vi "DOE Kitchen Data.vi"(6 "Data Logger Type":T1=enum."Agilent", 8 "Error In":errorcluster, 10 "Extra Data":dbl[](array[numeric]), 11 "Kitchen Input":T2) -> (0 "Error Out":errorcluster, 1 "Kitchen DBL Data":dbl[](array[numeric]), 2 "Kitchen Cluster":T2, 3 "Kitchen Analog Data":string[][](array[string]))   [LabVIEW 2018]
uses:
  Type Definitions/DOE Kitchen Control.ctl
  Type Definitions/DOE Data Logger Type.ctl
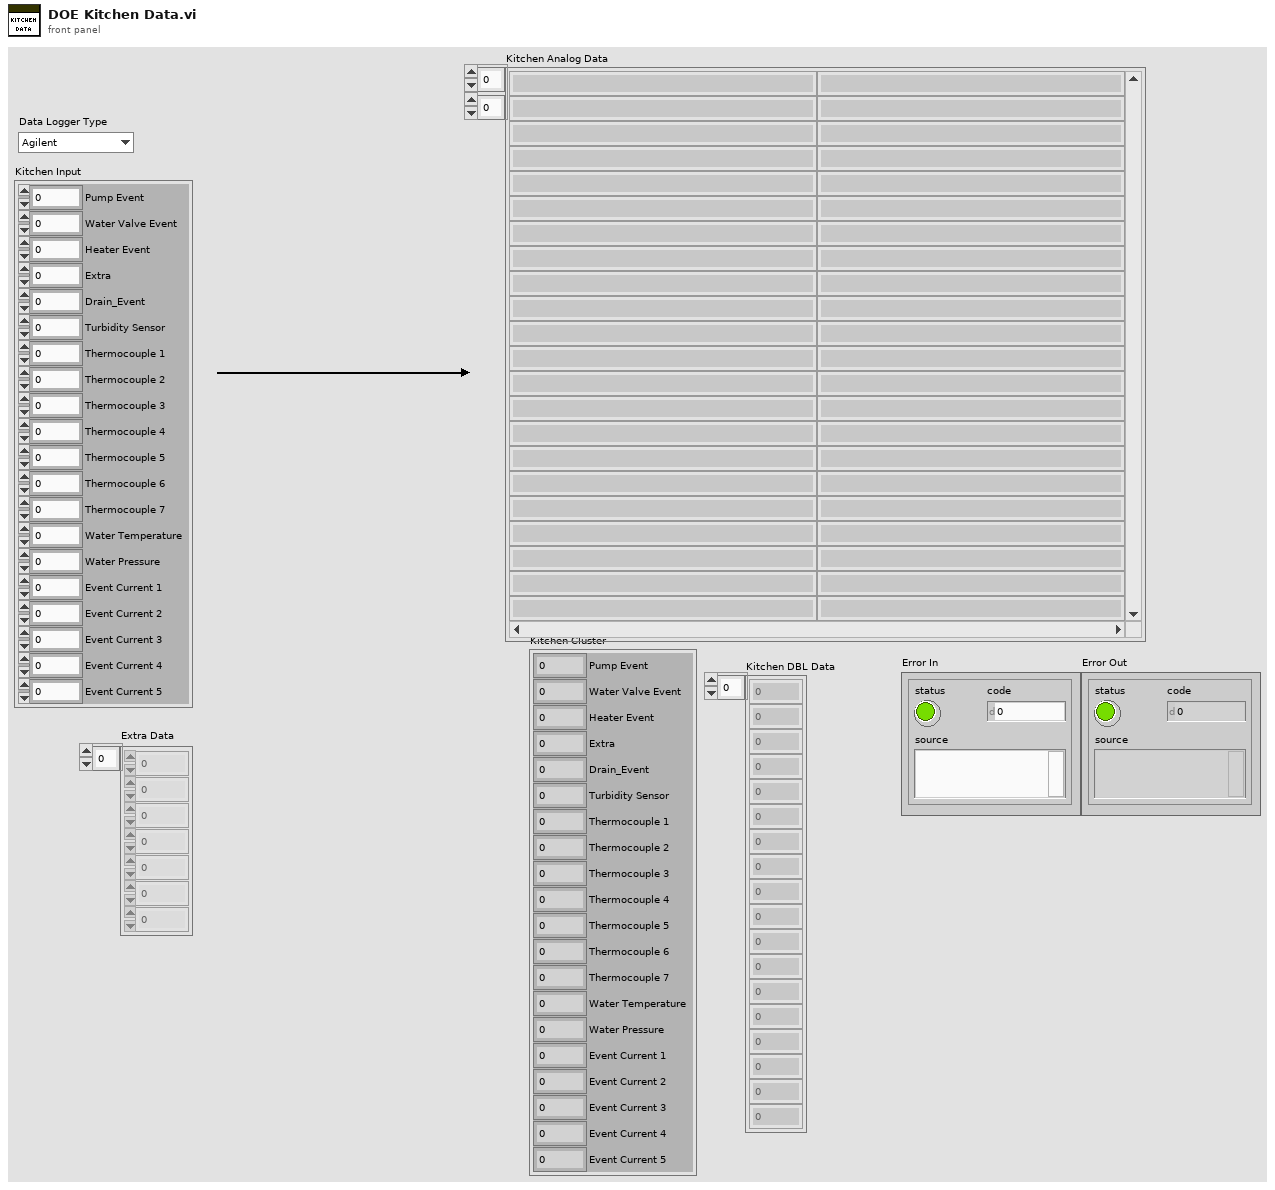
[diagram p1: front panel]
types:
  T1 = typedef "DOE Data Logger Type.ctl" = enum16{"MW100", "Agilent", "Agilent_Laurel_DC_Clamp"}
  T2 = typedef "DOE Kitchen Control.ctl" = cluster{"Drain_Event":i16, "Pump Event":i16, "Water Valve Event":i16, "Heater Event":i16, "Extra":i16, "Turbidity Sensor":dbl, "Thermocouple 1":dbl, "Thermocouple 2":dbl, "Thermocouple 3":dbl, "Thermocouple 4":dbl, "Thermocouple 5":dbl, "Thermocouple 6":dbl, "Water Temperature":dbl, "Water Pressure":dbl, "Event Current 1":dbl, "Event Current 2":dbl, "Event Current 3":dbl, "Event Current 4":dbl, "Event Current 5":dbl, "Thermocouple 7":dbl}
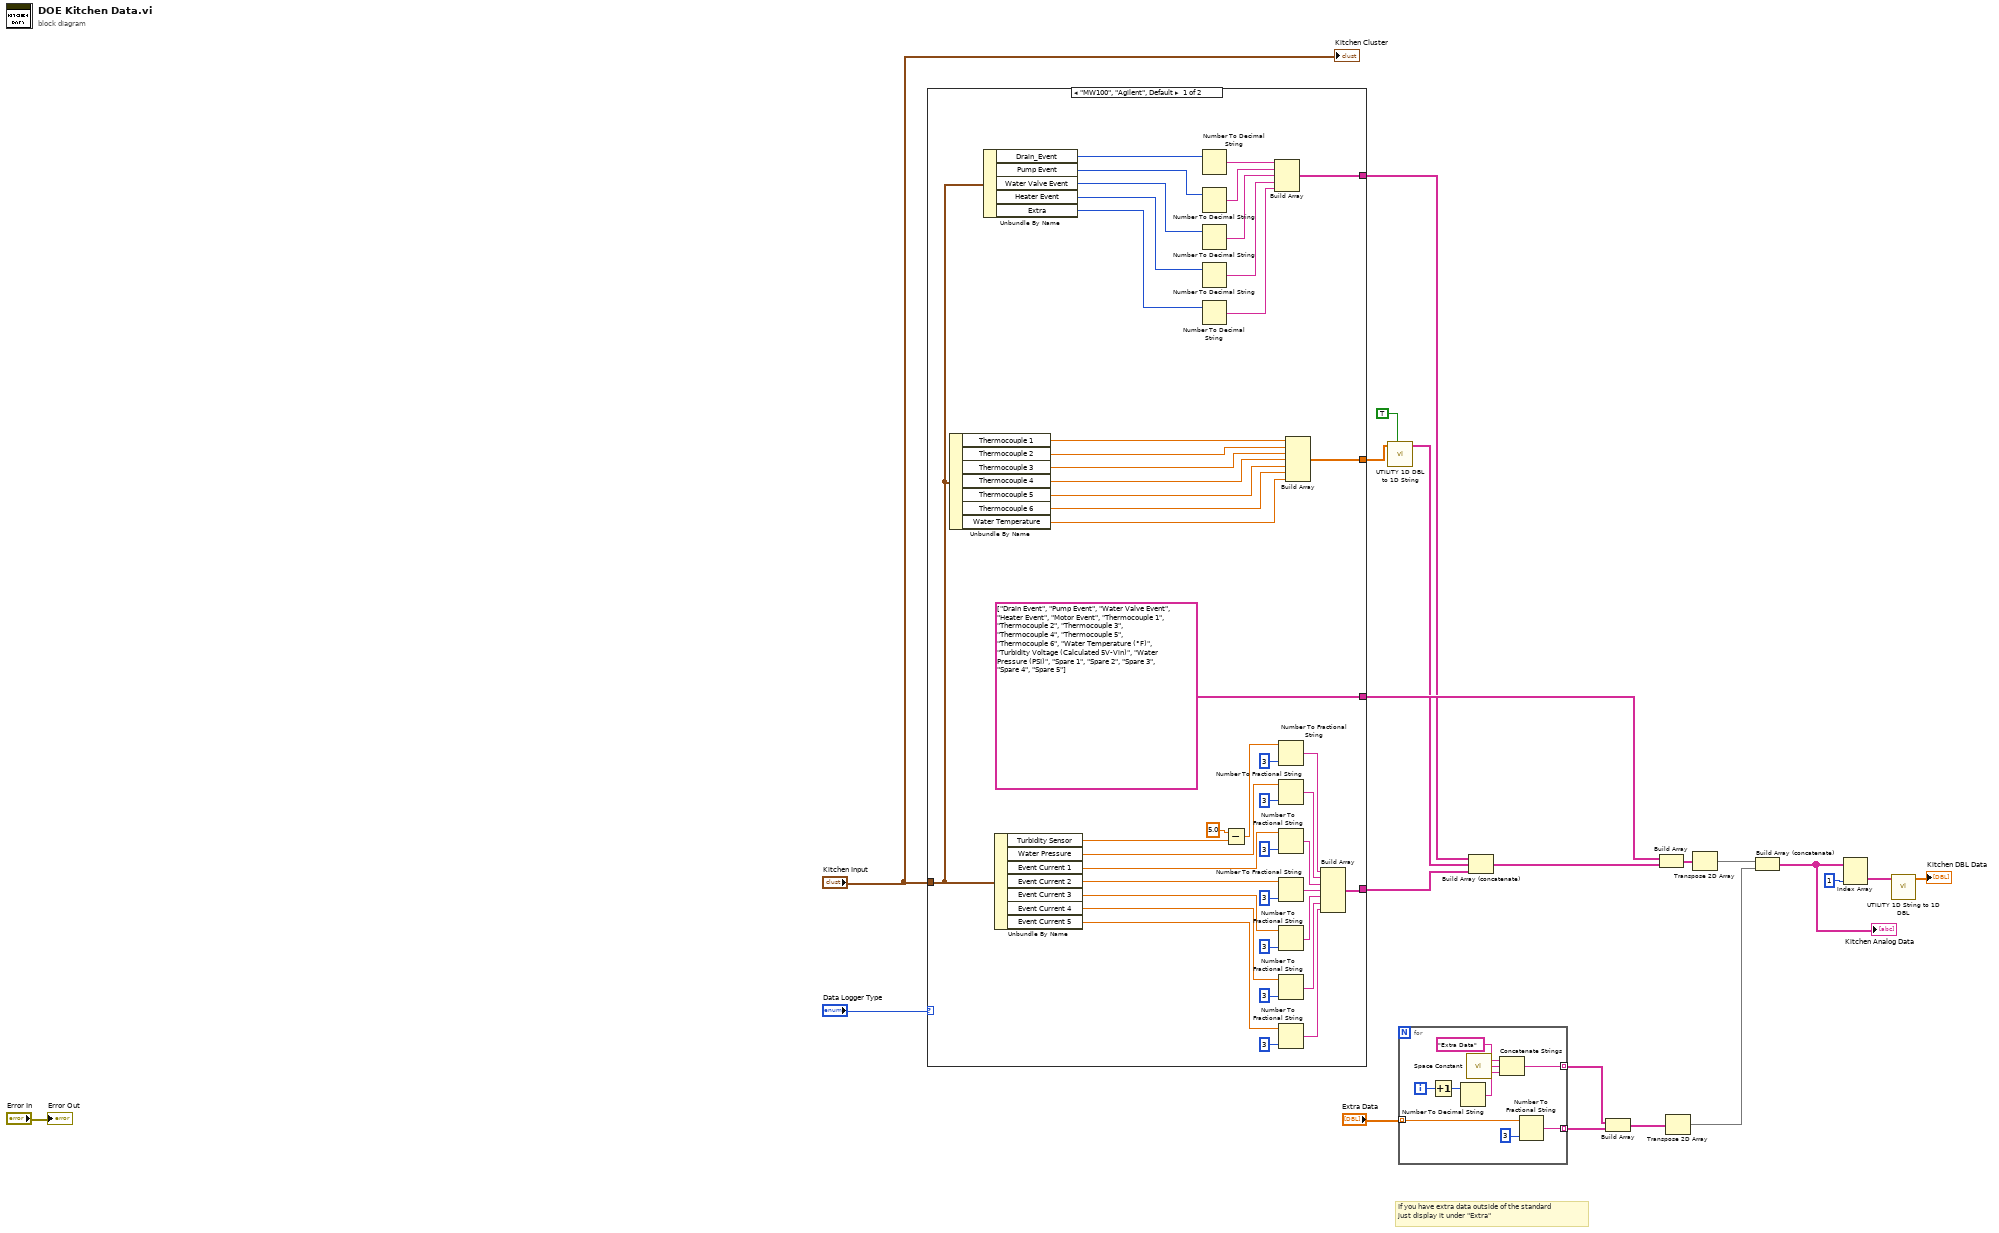
[diagram p0: block diagram]
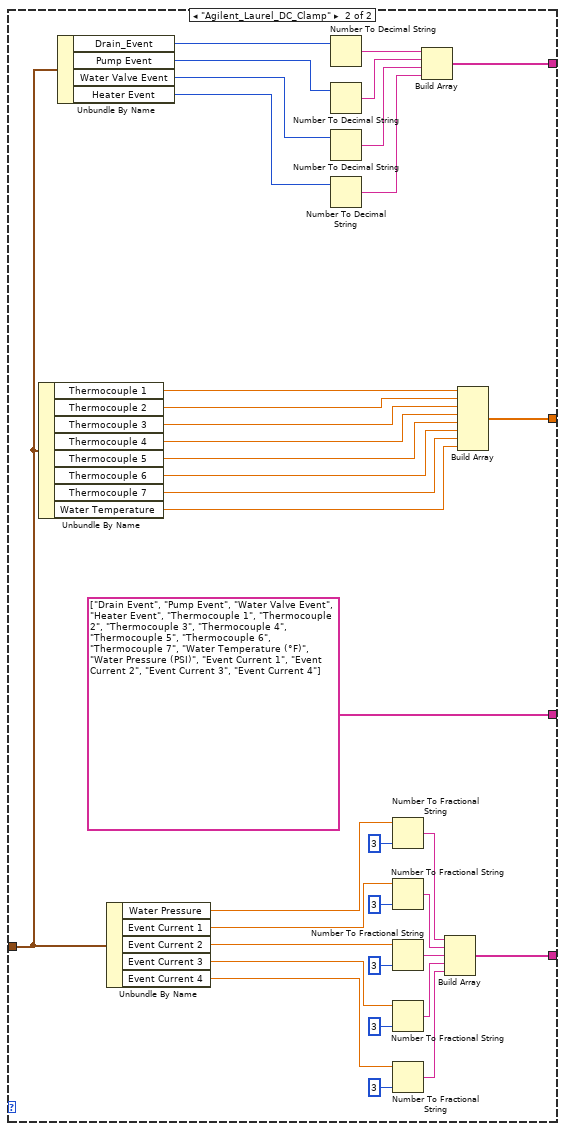
[diagram p2: hidden frame]
diagram:
  # "If you have extra data outside of the standard\njust display it under \"Extra\""
  n1 = case shown="\"MW100\", \"Agilent\", Default" "Data Logger Type" {
    tunnel: "Kitchen Input" -> [w23 w69]
    tunnel: [w43 w86] -> w17
    tunnel: [string[] ["Drain Event", "Pump Event", "Water Valve Event", "Heater Event", "Motor Event", "Thermocouple 1", "Thermocouple 2", "Thermocouple 3", "Thermocouple 4", "Thermocouple 5", "Thermocouple 6", "Water Temperature (°F)", "Turbidity Voltage (Calculated 5V-Vin)", "Water Pressure (PSI)", "Spare 1", "Spare 2", "Spare 3", "Spare 4", "Spare 5"] string[] ["Drain Event", "Pump Event", "Water Valve Event", "Heater Event", "Thermocouple 1", "Thermocouple 2", "Thermocouple 3", "Thermocouple 4", "Thermocouple 5", "Thermocouple 6", "Thermocouple 7", "Water Temperature (°F)", "Water Pressure (PSI)", "Event Current 1", "Event Current 2", "Event Current 3", "Event Current 4"]] -> w15
    tunnel: [w24 w68] -> w4
    tunnel: [w22 w67] -> w2
    frame "MW100", "Agilent", Default {
      n2 = Unbundle By Name(w23) -> ("Thermocouple 1"=w35:dbl, "Thermocouple 2"=w36:dbl, "Thermocouple 3"=w37:dbl, "Thermocouple 4"=w38:dbl, "Thermocouple 5"=w39:dbl, "Thermocouple 6"=w40:dbl, "Water Temperature"=w41:dbl)
      n3 = Unbundle By Name(w23) -> ("Drain_Event"=w25:i16, "Pump Event"=w26:i16, "Water Valve Event"=w27:i16, "Heater Event"=w28:i16, "Extra"=w29:i16)
      n4 = Unbundle By Name(w23) -> ("Turbidity Sensor"=w53:dbl, "Water Pressure"=w66:dbl, "Event Current 1"=w59:dbl, "Event Current 2"=w58:dbl, "Event Current 3"=w57:dbl, "Event Current 4"=w56:dbl, "Event Current 5"=w54:dbl)
      n5 = Number To Decimal String(number=w25) -> (decimal integer string=w30:string)  [unwired: 1 in]
      n6 = Number To Decimal String(number=w26) -> (decimal integer string=w31:string)  [unwired: 1 in]
      n7 = Number To Decimal String(number=w27) -> (decimal integer string=w32:string)  [unwired: 1 in]
      n8 = Number To Decimal String(number=w28) -> (decimal integer string=w33:string)  [unwired: 1 in]
      n9 = Number To Decimal String(number=w29) -> (decimal integer string=w34:string)  [unwired: 1 in]
      n10 = Subtract(x=5.0, y=w53) -> (x-y=w51:dbl)
      n11 = Build Array(w30, w31, w32, w33, w34) -> (w24:string[])
      n12 = Number To Fractional String(number=w51, precision (6)=i16 3) -> (F-format string=w50:string)  [unwired: 2 in]
      n13 = Number To Fractional String(number=w66, precision (6)=i16 3) -> (F-format string=w49:string)  [unwired: 2 in]
      n14 = Number To Fractional String(number=w59, precision (6)=i16 3) -> (F-format string=w48:string)  [unwired: 2 in]
      n15 = Number To Fractional String(number=w58, precision (6)=i16 3) -> (F-format string=w47:string)  [unwired: 2 in]
      n16 = Number To Fractional String(number=w57, precision (6)=i16 3) -> (F-format string=w46:string)  [unwired: 2 in]
      n17 = Number To Fractional String(number=w56, precision (6)=i16 3) -> (F-format string=w45:string)  [unwired: 2 in]
      n18 = Number To Fractional String(number=w54, precision (6)=i16 3) -> (F-format string=w44:string)  [unwired: 2 in]
      n19 = Build Array(w35, w36, w37, w38, w39, w40, w41) -> (w22:dbl[])
      n20 = Build Array(w50, w49, w48, w47, w46, w45, w44) -> (w43:string[])
    }
    frame "Agilent_Laurel_DC_Clamp" {
      n21 = Unbundle By Name(w69) -> ("Thermocouple 1"=w79:dbl, "Thermocouple 2"=w80:dbl, "Thermocouple 3"=w81:dbl, "Thermocouple 4"=w82:dbl, "Thermocouple 5"=w83:dbl, "Thermocouple 6"=w84:dbl, "Thermocouple 7"=w78:dbl, "Water Temperature"=w85:dbl)
      n22 = Unbundle By Name(w69) -> ("Drain_Event"=w70:i16, "Pump Event"=w71:i16, "Water Valve Event"=w72:i16, "Heater Event"=w73:i16)
      n23 = Unbundle By Name(w69) -> ("Water Pressure"=w102:dbl, "Event Current 1"=w96:dbl, "Event Current 2"=w95:dbl, "Event Current 3"=w94:dbl, "Event Current 4"=w93:dbl)
      n24 = Number To Decimal String(number=w70) -> (decimal integer string=w74:string)  [unwired: 1 in]
      n25 = Number To Decimal String(number=w71) -> (decimal integer string=w75:string)  [unwired: 1 in]
      n26 = Number To Decimal String(number=w72) -> (decimal integer string=w76:string)  [unwired: 1 in]
      n27 = Number To Decimal String(number=w73) -> (decimal integer string=w77:string)  [unwired: 1 in]
      n28 = Number To Fractional String(number=w102, precision (6)=i16 3) -> (F-format string=w92:string)  [unwired: 2 in]
      n29 = Number To Fractional String(number=w96, precision (6)=i16 3) -> (F-format string=w91:string)  [unwired: 2 in]
      n30 = Number To Fractional String(number=w95, precision (6)=i16 3) -> (F-format string=w90:string)  [unwired: 2 in]
      n31 = Number To Fractional String(number=w94, precision (6)=i16 3) -> (F-format string=w89:string)  [unwired: 2 in]
      n32 = Number To Fractional String(number=w93, precision (6)=i16 3) -> (F-format string=w88:string)  [unwired: 2 in]
      n33 = Build Array(w74, w75, w76, w77) -> (w68:string[])
      n34 = Build Array(w92, w91, w90, w89, w88) -> (w86:string[])
      n35 = Build Array(w79, w80, w81, w82, w83, w84, w78, w85) -> (w67:dbl[])
    }
  }
  n36 = call "UTILITY 1D DBL to 1D String.vi"("DBL?"=TRUE, "1D DBL"=w2) -> ("1D String"=w1:string[])  [unwired: 9 in]
  n37 = for {
    tunnel: "Extra Data" -> [w106] mode=indexing
    tunnel: [w104] -> w10 mode=indexing
    tunnel: [w103] -> w11 mode=indexing
    i -> [w111]
    n38 = Increment(x=w111) -> (x+1=w108:i32)
    n39 = Number To Decimal String(number=w108) -> (decimal integer string=w107:string)  [unwired: 1 in]
    n40 = call <vilib>:"Space Constant.vi"() -> ("String"=w109:string)
    n41 = Concatenate Strings("Extra Data", w109, w107) -> (w103:string)
    n42 = Number To Fractional String(number=w106, precision (6)=i16 3) -> (F-format string=w104:string)  [unwired: 2 in]
  }
  n43 = Build Array (concatenate)(w4, w1, w17) -> (w21:string[])
  n44 = Build Array(w11, w10) -> (w9:string[][])
  n45 = Build Array(w15, w21) -> (w20:string[][])
  n46 = Transpose 2D Array(2D array=w9) -> (transposed array=w7:string[][])
  n47 = Transpose 2D Array(2D array=w20) -> (transposed array=w8:string[][])
  n48 = Build Array (concatenate)(w8, w7) -> (w6:string[][])
  "Kitchen Analog Data" <- w6
  n49 = Index Array(array=w6, index (col)=1 ("disabled index (col)")) -> (element=w14:string[])  [unwired: 1 in]
  n50 = call "UTILITY 1D String to 1D DBL.vi"("Save Data"=w14) -> ("DBL"=→"Kitchen DBL Data":dbl[])  [unwired: 10 in]
  "Kitchen Cluster" <- "Kitchen Input"
  "Error Out" <- "Error In"
